vi "Create Arbitrary Waveform For Two Channels.vi"(6 "Timeout (10000 ms)":i32=10000, 7 "Arbitrary Data Format (1: ABAB)":i32(ring)=1 items=["AABB"=1, "ABAB"=2], 8 "error in (no error)":errorcluster, 9 "Arbitrary Waveform Data":dbl[](array[numeric]), 10 "Arbitrary Waveform Name (ARB1)":string="ARB1", 11 "VISA resource name":refnum<visa-resource-name>) -> (0 "error out":errorcluster, 3 "VISA resource name out":refnum<visa-resource-name>)   [LabVIEW 2016, in "Agilent 3352X Series.lvlib"]
doc: "Creates and saves arbitrary (user-defined) waveforms in volatile memory. \nThe data array specified contains two channles of data.\n\n<B>Note</B>: \n(1) You must specify at least 14 numbers for waveform data\n(2) Call Configure Arbitrary Waveform VI to activate it and change the settings.\n(3) Volatile memory will be cleared when you turn off your instrument or call Load State.vi.\n(4) You can store current loaded arb to non-volatile memory using Store Arbitrary Waveform.vi\n(5) This function only works for 33522B with optional IQ Player."
uses:
  Agilent 3352X Series.lvlib
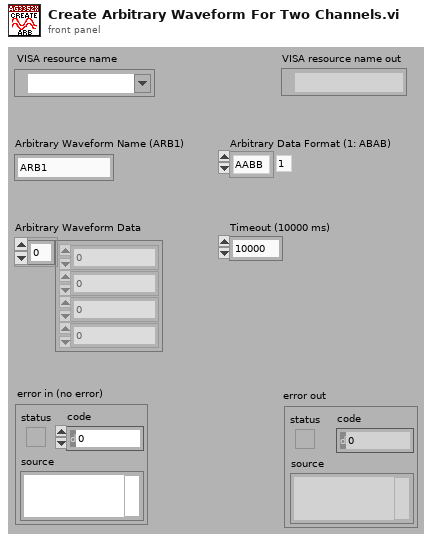
[diagram p1: front panel]
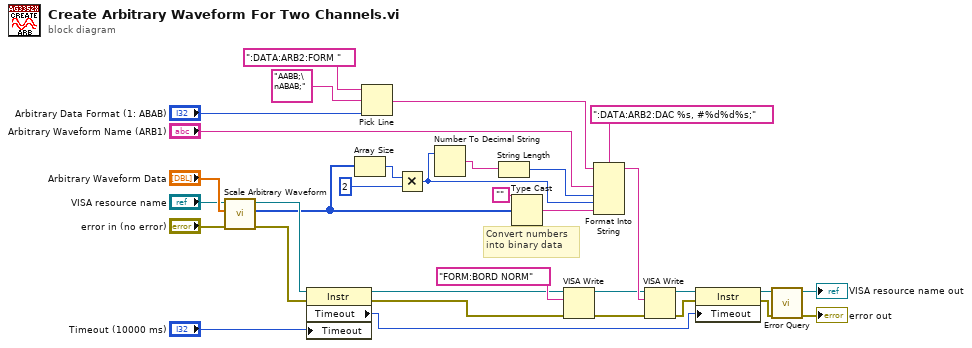
[diagram p0: block diagram]
diagram:
  # "Convert numbers\ninto binary data"
  n1 = call "Scale Arbitrary Waveform.vi"("error in (no error)"="error in (no error)", "Arbitrary Waveform Data"="Arbitrary Waveform Data", "VISA resource name"="VISA resource name") -> ("error out"=w20:errorcluster, "Scaled Arbitrary Waveform Data"=w12:i16[], "VISA resource name out"=w22:refnum<visa-resource-name>)  [unwired: 6 out]
  n2 = property on="Property Node" class="Instr"(reference=w22, error in=w20, "Timeout"="Timeout (10000 ms)") -> (reference out=w18:refnum<visa-resource-name>, error out=w17:errorcluster, "Timeout"=w30:u32)
  n3 = Array Size(array=w12) -> (size(s)=w11:i32)
  n4 = Pick Line(string ("")=":DATA:ARB2:FORM " ("multi-line string"), multi-line string="AABB;\nABAB;", line index="Arbitrary Data Format (1: ABAB)") -> (output string=w1:string)
  n5 = Multiply(x=w11, y=2 ("size(s)")) -> (x*y=w3:i32)
  n6 = Number To Decimal String(number=w3) -> (decimal integer string=w9:string)  [unwired: 1 out]
  n7 = String Length(string=w9) -> (length=w5:i32)
  n8 = Type Cast(type="" ("Empty String Constant"), x=w12) -> (*(type *) &x=w4:string)
  n9 = VISA Write(VISA resource name=w18, write buffer="FORM:BORD NORM", error in (no error)=w17) -> (VISA resource name out=w16:refnum<visa-resource-name>, error out=w15:errorcluster)  [unwired: 1 out]
  n10 = Format Into String(format string=":DATA:ARB2:DAC %s, #%d%d%s;", initial string=w1, "Arbitrary Waveform Name (ARB1)", w5, w3, w4) -> (resulting string=w32:string)  [unwired: 1 in, 1 out]
  n11 = VISA Write(VISA resource name=w16, write buffer=w32, error in (no error)=w15) -> (VISA resource name out=w27:refnum<visa-resource-name>, error out=w29:errorcluster)  [unwired: 1 out]
  n12 = property on="Property Node" class="Instr"(reference=w27, error in=w29, "Timeout"=w30) -> (reference out=w25:refnum<visa-resource-name>, error out=w28:errorcluster)
  n13 = call "Error Query.vi"("error in (no error)"=w28, "VISA resource name"=w25) -> ("error out"=→"error out":errorcluster, "VISA resource name out"=→"VISA resource name out":refnum<visa-resource-name>)  [unwired: 8 out]
